vi "Window Memory write - Host.vi"(8 "error in":errorcluster, 11 "FPGA VI Reference In":refnum<k20>) -> (0 "FPGA VI Reference Out":refnum<k20>, 3 "error out":errorcluster, 6 "Write memory Window complete":bool)   [LabVIEW 2014]
uses:
  <vilib>/Utility/error.llb/Error Cluster From Error Code.vi
  <vilib>/RVI Host/nirviSupport.llb/nirviErrorClusterFromErrorCode.vi
  <vilib>/rvi/errors/niLvFpgaAdjustHostInterfaceError.vi
  <vilib>/rvi/interface/nirviMethod/nirviMethod.xnode
  <vilib>/rvi/interface/nirviMethod/StockFPGA_InlinedMethodWaitForSingleIRQ.vi
  <vilib>/FPGAPlugInAG/Dynamic/niLvFpga_WaitOnIrq_Dynamic.vi
  <vilib>/FPGAPlugInAG/Dynamic/niLvFpga_AcknowledgeIrq_Dynamic.vi
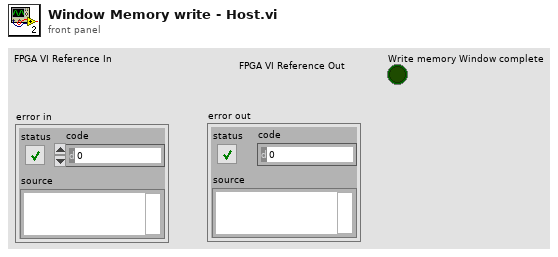
[diagram p1: front panel]
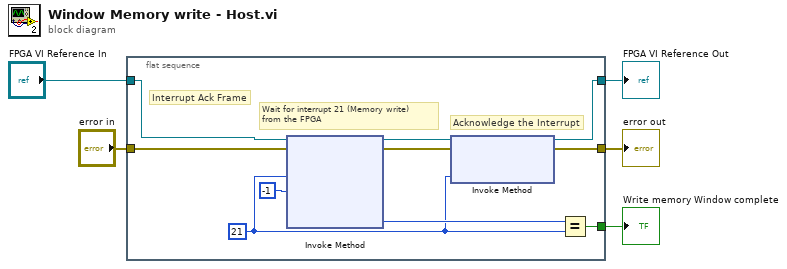
[diagram p0: block diagram]
diagram:
  n1 = flat-sequence {
    tunnel: [w11] -> w3
    tunnel: [w12] -> w5
    tunnel: [w8] -> w4
    tunnel: "FPGA VI Reference In" -> [w7]
    tunnel: "error in" -> [w6]
    frame #0 {
      w9 = 21 ("IRQ Number(s)")
      # "Acknowledge the Interrupt"
      # "Wait for interrupt 21 (Memory write)\nfrom the FPGA"
      # "Interrupt Ack Frame"
      n2 = xnode "Invoke Method"("FPGA VI Reference In"=w7, "error in"=w6, "IRQ Number(s)"=w9, "Timeout (ms)"=-1) -> ("FPGA VI Reference Out"=w13:refnum<k20>, "error out"=w14:errorcluster, "IRQ(s) Asserted"=w10:i32)  [unwired: 1 out]
      n3 = xnode "Invoke Method"("FPGA VI Reference In"=w13, "error in"=w14, "IRQ Number(s)"=w9) -> ("FPGA VI Reference Out"=w11:refnum<k20>, "error out"=w12:errorcluster)
      n4 = Equal?(x=w10, y=w9) -> (x = y?=w8:bool)
    }
  }
  "error out" <- w5
  "Write memory Window complete" <- w4
  "FPGA VI Reference Out" <- w3
